vi "detector_get_data_dimensions.vi"(8 "error in (no error)":errorcluster, 11 "lightfield_class in":refnum<class "lightfield_class.lvclass">) -> (0 "error out":errorcluster, 1 "data_type":T1, 2 "dims":u32[](array[numeric]), 3 "lightfield_class out":refnum<class "lightfield_class.lvclass">)   [LabVIEW 2015, in "lightfield_class.lvclass"]
uses:
  lightfield_class.lvclass
  detector/data_types_tdef.ctl
  lightfield_class.lvclass/lightfield_class.ctl
  lightfield-automation-labview/LightField Automation.lvclass
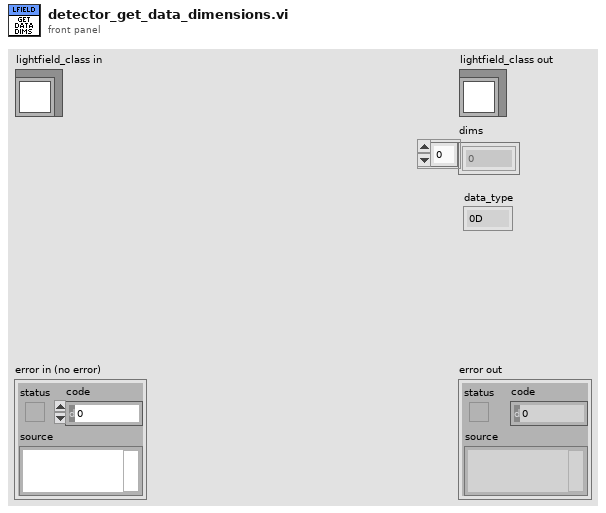
[diagram p1: front panel]
types:
  T1 = typedef "data_types_tdef.ctl" = enum16{"0D", "1D", "2D"}
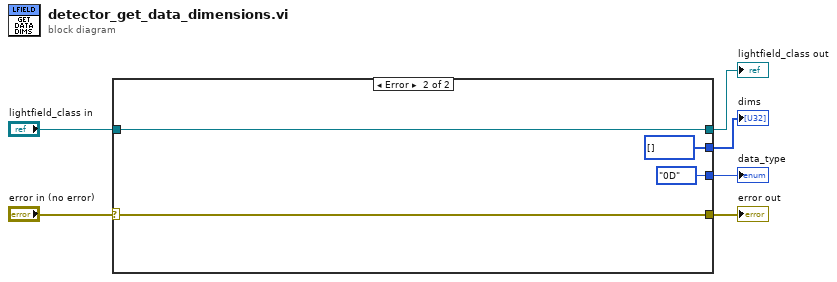
[diagram p0: block diagram]
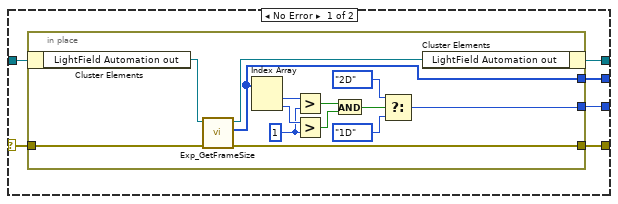
[diagram p2: hidden frame]
diagram:
  n1 = case shown="Error" "error in (no error)" {
    selector: "error in (no error)" -> [w11 w28]
    tunnel: "lightfield_class in" -> [w12 w30]
    tunnel: [w10 w28] -> w4
    tunnel: [w9 i32[] [] ("frame_size")] -> w3
    tunnel: [w8 w30] -> w2
    tunnel: [w7 data_types_tdef."0D" ("data_type")] -> w1
    frame No Error {
      n2 = in-place {
        in-place-border: w11 -> [w25]
        in-place-border: [w24] -> w10
        in-place-border: [w22] -> w9
        in-place-border: [w13] -> w7
        w19 = 1 ("y")
        n3 = in-place-cluster #1(w12) -> ("LightField Automation out"=w26:refnum<class "LightField Automation.lvclass">)
        n4 = call "Exp_GetFrameSize.vi"("error in (no error)"=w25, "LightField Automation in"=w26) -> ("error out"=w24:errorcluster, "frame_size"=w22:i32[], "LightField Automation out"=w23:refnum<class "LightField Automation.lvclass">)  [unwired: 7 in]
        n5 = Index Array(array=w22) -> (element #1=w21:i32, element #2=w20:i32)  [unwired: 2 in]
        n6 = Greater?(x=w21, y=w19) -> (0:w17:bool)
        n7 = Greater?(x=w20, y=w19) -> (0:w18:bool)
        n8 = And(x=w17, y=w18) -> (x .and. y?=w14:bool)
        n9 = Select(t=data_types_tdef."2D" ("data_type"), s=w14, f=data_types_tdef."1D" ("data_type")) -> (s? t:f=w13:T1)
        n10 = in-place-cluster #1("LightField Automation out"=w23) -> (w8:refnum<class "lightfield_class.lvclass">)
      }
    }
    frame Error {
    }
  }
  "error out" <- w4
  "lightfield_class out" <- w2
  "dims" <- w3
  "data_type" <- w1
